vi "_GetHelp 1.vi"(0 "XRef":T16, 1 "Point":T15, 2 "State In":T14) -> (14 "Standard Help Info":T12, 15 "Detailed Help Info":T9, 16 "Subitem Help Info":T3, 17 "Use Detailed Help?":T2, 18 "Use Subitem Help?":T2, 19 "Fatal Error Out":T1)   [LabVIEW 2014, in "JKISM++ DebugTool.xnode"]
doc: "Launch VI Package Manager to discover and install LabVIEW add-ons from the LabVIEW Tools Network. Package your own reusable code and share it with others."
uses:
  JKISM++ DebugTool.xnode
  <vilib>/XNodeSupport/XNodeXNodeRef.ctl
  <vilib>/XNodeSupport/XNodePoint.ctl
  <vilib>/XNodeSupport/XNodeInt.ctl
  _State 1.ctl
  <vilib>/XNodeSupport/XNodeStandardHelpInfo.ctl
  <vilib>/XNodeSupport/XNodeString.ctl
  <vilib>/XNodeSupport/XNodePath.ctl
  <vilib>/XNodeSupport/XNodeDetailedHelpInfo.ctl
  <vilib>/XNodeSupport/XNodeImage.ctl
  <vilib>/XNodeSupport/XNodeRect32.ctl
  <vilib>/XNodeSupport/XNodeTerms.ctl
  <vilib>/XNodeSupport/XNodeTerm.ctl
  <vilib>/XNodeSupport/XNodeVariant.ctl
  <vilib>/XNodeSupport/XNodeBool.ctl
  <vilib>/XNodeSupport/XNodeSubitemHelpInfo.ctl
  <vilib>/XNodeSupport/XNodeErrorCluster.ctl
  <vilib>/XNodeSupport/NI_XNodeSupport.lvlib
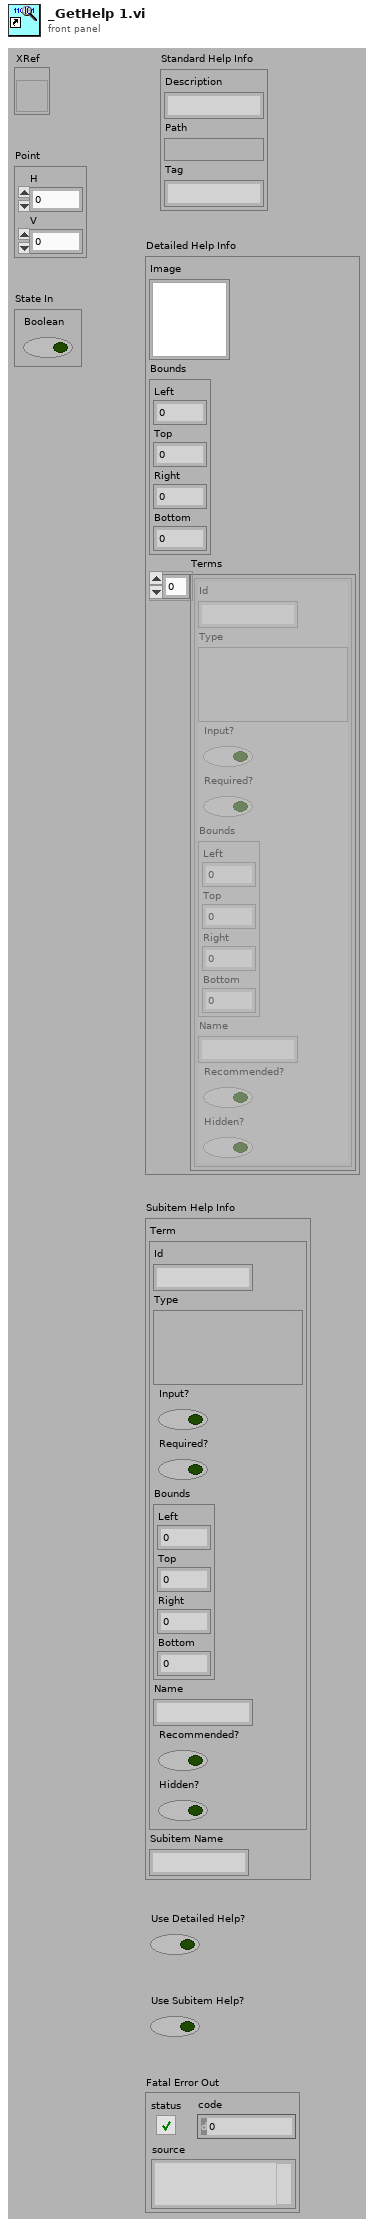
[diagram p1: front panel]
types:
  T1 = typedef "NI_XNodeSupport.lvlib/XNodeErrorCluster.ctl" = errorcluster
  T2 = typedef "NI_XNodeSupport.lvlib/XNodeBool.ctl" = bool
  T3 = typedef "NI_XNodeSupport.lvlib/XNodeSubitemHelpInfo.ctl" = cluster{"Term":T4, "Subitem Name":T5}
  T4 = typedef "NI_XNodeSupport.lvlib/XNodeTerm.ctl" = cluster{"Id":T5, "Type":T6, "Input?":T2, "Required?":T2, "Bounds":T7, "Name":T5, "Recommended?":T2, "Hidden?":T2}
  T5 = typedef "NI_XNodeSupport.lvlib/XNodeString.ctl" = string
  T6 = typedef "NI_XNodeSupport.lvlib/XNodeVariant.ctl" = variant
  T7 = typedef "NI_XNodeSupport.lvlib/XNodeRect32.ctl" = cluster{"Left":T8, "Top":T8, "Right":T8, "Bottom":T8}
  T8 = typedef "NI_XNodeSupport.lvlib/XNodeInt.ctl" = i32
  T9 = typedef "NI_XNodeSupport.lvlib/XNodeDetailedHelpInfo.ctl" = cluster{"Image":T10, "Bounds":T7, "Terms":T11}
  T10 = typedef "NI_XNodeSupport.lvlib/XNodeImage.ctl" = picture
  T11 = typedef "NI_XNodeSupport.lvlib/XNodeTerms.ctl" = T4[]
  T12 = typedef "NI_XNodeSupport.lvlib/XNodeStandardHelpInfo.ctl" = cluster{"Description":T5, "Path":T13, "Tag":T5}
  T13 = typedef "NI_XNodeSupport.lvlib/XNodePath.ctl" = path
  T14 = typedef "JKISM++ DebugTool.xnode/_State 1.ctl" = cluster{"Boolean":bool}
  T15 = typedef "NI_XNodeSupport.lvlib/XNodePoint.ctl" = cluster{"H":T8, "V":T8}
  T16 = typedef "NI_XNodeSupport.lvlib/XNodeXNodeRef.ctl" = refnum<vi>
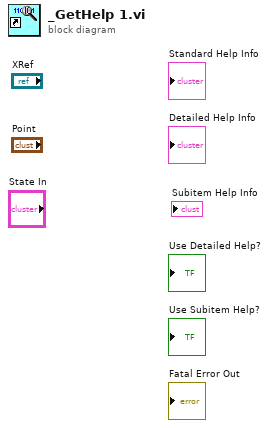
[diagram p0: block diagram]
diagram:
